vi "Test.vi"() -> ()   [LabVIEW 2015]
panel:
  in  "运行按钮":bool(xcontrol)
  out "数字(0-1)":dbl
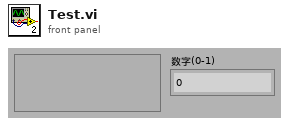
[diagram p1: front panel]
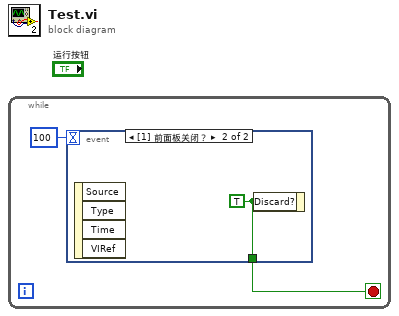
[diagram p0: block diagram]
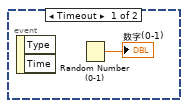
[diagram p2: hidden frame]
diagram:
  n1 = while {
    stop <- w1 stop-if-true
    n2 = event shown="[1] 前面板关闭？" {
      selector: _ -> [_ _]
      dyn-events: _ -> [_ _]
      timeout: 100 -> [_ _]
      tunnel: [_ w4] -> w1
      event Timeout {
        n3 = event-data() -> ()  [unwired: 1 in, 2 out]
        n4 = Random Number (0-1)() -> (number: 0 to 1=→"数字(0-1)":dbl)
      }
      event Panel Close? {
        w4 = TRUE ("放弃？")
        n5 = event-data() -> ()  [unwired: 1 in, 4 out]
        n6 = event-data("Discard?"=w4) -> ()  [unwired: 1 in, 1 out]
      }
    }
  }
